vi "Write modbus.vi"(10 "Modbus Master":refnum<class "Modbus Master.lvclass">, 11 "MB_MODULE in":refnum<class "MB_MODULE.lvclass">) -> (3 "MB_MODULE out":refnum<class "MB_MODULE.lvclass">)   [LabVIEW 2019, in "MB_MODULE.lvclass"]
uses:
  MB_MODULE.lvclass
  <vilib>/NI/Modbus Library/API/Master/Modbus Master.lvclass
  MB_MODULE.lvclass/MB_MODULE.ctl
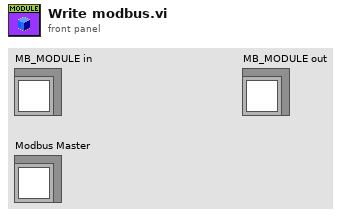
[diagram p1: front panel]
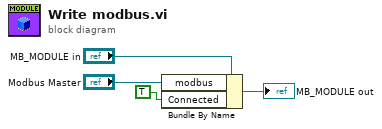
[diagram p0: block diagram]
diagram:
  n1 = Bundle By Name(cluster="MB_MODULE in", "modbus"="Modbus Master", "Connected"=TRUE) -> (→"MB_MODULE out":refnum<class "MB_MODULE.lvclass">)
